vi "StepRealtime_IP6.vi"() -> ()   [LabVIEW 2011]
doc: "This VI was generated automatically using the FPGA Wizard. You can modify the VI normally."
uses:
  <vilib>/Platform/TimedLoop/XDataNode/timing_clust.ctl
  <vilib>/Platform/TimedLoop/XDataNode/nitl_modes.ctl
  <vilib>/Platform/TimedLoop/XDataNode/wakeup.ctl
  <vilib>/FPGAPlugInAG/sbRIO-9632/niLvFpga_Open_sbRIO-9632.vi
  <vilib>/rvi/interface/common/dynamic/niFpgaDynamicAddResources.vi
  <vilib>/FPGAPlugInAG/Dynamic/niLvFpga_Reset_Dynamic.vi
  <vilib>/FPGAPlugInAG/Dynamic/niLvFpga_Run_Dynamic.vi
  <vilib>/Utility/error.llb/Error Cluster From Error Code.vi
  <vilib>/rvi/errors/niLvFpgaAdjustHostInterfaceError.vi
  <vilib>/FPGAPlugInAG/Dynamic/niLvFpga_Close_Dynamic.vi
  <vilib>/rvi/interface/nirviOpenFPGA/nirviOpenFPGA.xnode
  FPGA Bitfiles/PPDControlLab3_FPGATarget_IP6.lvbitx
  <vilib>/rvi/interface/nirviMethod/nirviMethod.xnode
  <vilib>/Platform/TimedLoop/XDataNode/XDataNode.xnode
  <vilib>/rvi/interface/nirviReadWriteControl/nirviReadWriteControl.xnode
  <vilib>/rvi/interface/nirviCloseFPGA/nirviCloseFPGA.xnode
  SysIDRealtime.lvlib
  <vilib>/rvi/interface/Simulation/niFpgaSimulationCallBeginRW.vi
  <vilib>/Platform/TimedLoop/XDataNode/XDNodeRunTimeDep.lvlib
  NiFpgaLv.dll
panel:
  out "Ratio":fxp<+/-,32,7>
  in  "Gain":fxp<+/-,32,7>=0.006999999284744263
  in  "Radio Buttons":enum32{"Radio Selection 1", "Radio Selection 2"}(radio)
  in  "OK Button":bool
  out "Step Response":dynamicdata(graph)=[{"t0"=timestamp(0 s since 1904-01-01), "dt"=1.0, "Y"=array[2048 elements]}, {"t0"=timestamp(0 s since 1904-01-01), "dt"=1.0, "Y"=array[2048 elements]}, {"t0"=timestamp(0 s since 1904-01-01), "dt"=1.0, "Y"=array[2048 elements]}]
  in  "samples":i32=2048
  in  "Reference":i32=100000
  in  "Quad Reset":bool=TRUE
  in  "DGain":fxp<+/-,32,7>
  in  "PGain":fxp<+/-,32,7>
  out "Amp In":dbl[](graph)
  out "Amp Cpmmand":fxp<+/-,20,5>
  out "Iteration Duration":i64
  out "Position":i32[](graph)
  in  "Control Rate (ticks)":u32=10000
  in  "Period (us)":i64=1000
  out "Finished Late? [i-1]":bool
  out "quad saved (Port0/DIO0,Port0/DIO1)":cluster{"Position":i32, "Index Count":u16}
  out "quad pos (Port0/DIO0,Port0/DIO1)":i32
  out "Late? Latched":bool
  in  "Local Stop 0":bool
  in  "Start 0":bool
  in  "Loop Rate (Hz)":dbl=100000.0
  out "Calculated Rate (Hz)":dbl
  out "error out":errorcluster
  in  "Global Stop":bool
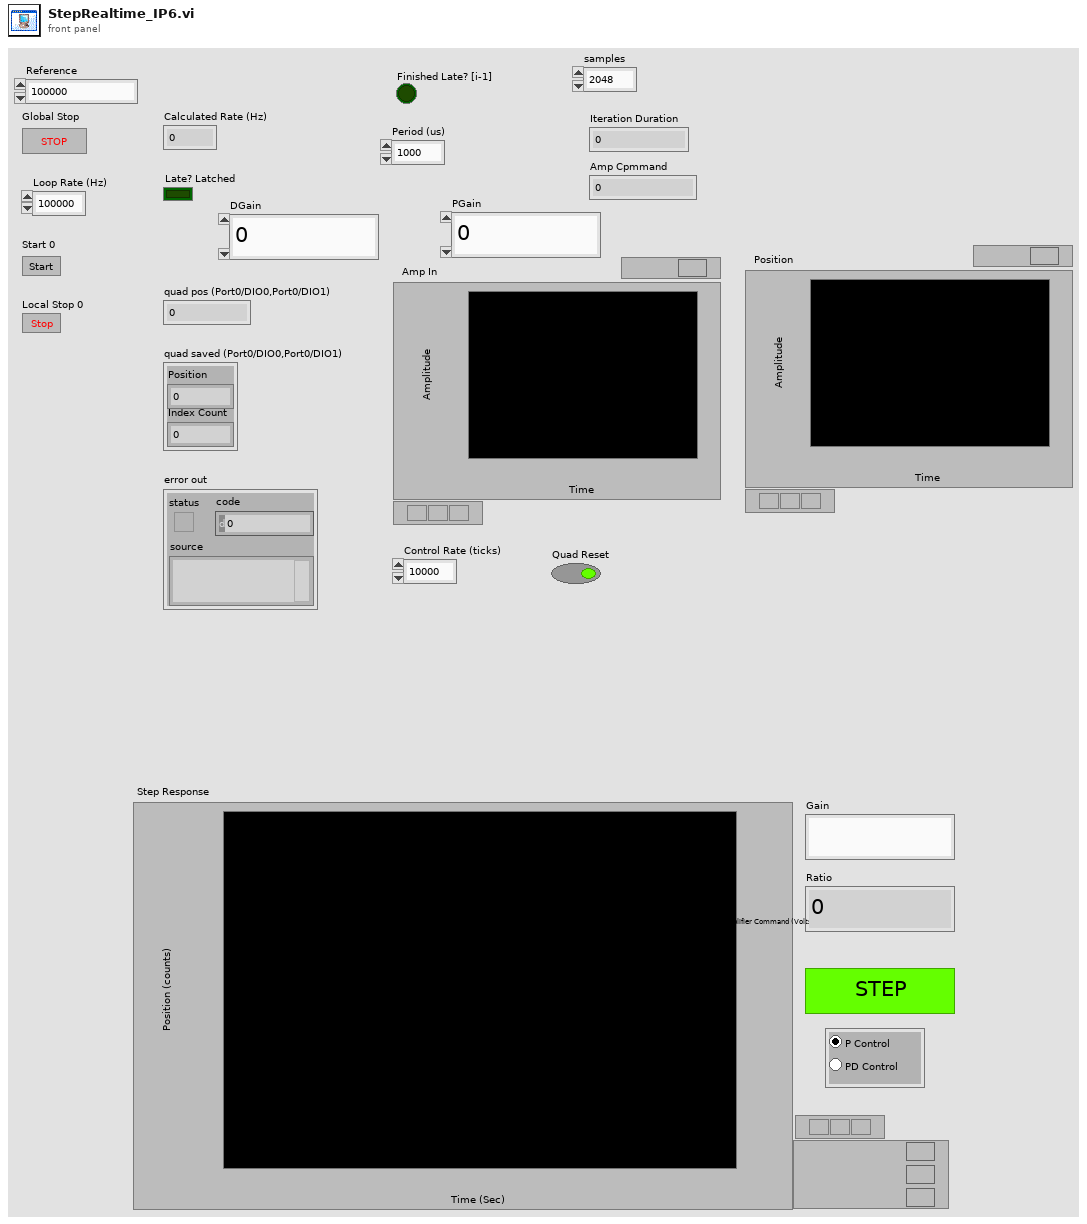
[diagram p1: front panel]
types:
  T1 = typedef "XDNodeRunTimeDep.lvlib/timing_clust.ctl" = cluster{"Expected End [f-1]":u64, "Actual End [f-1]":u64, "Finished Late? [f-1]":bool, "Expected End [i-1]":u64, "Actual End [i-1]":u64, "Finished Late? [i-1]":bool, "Expected Start [i]":u64, "Actual Start [i]":u64, "Expected Start [f]":u64, "Actual Start [f]":u64, "Source Name":string, "Structure Name":string, "Period":i64, "Deadline":i64, "Offset":i64, "Start":i64, "Priority":i32, "Timeout":i32, "Mode":T2, "Wakeup Reason":T3, "Error":errorcluster, "Source Type":string, "Secondary Source Type":string, "Global End Time":u64, "Global Start Time":u64, "Frame Duration":u64, "Iteration Duration":u64, "Assigned CPU":i32, "I/O Scan Engine Mode":u32}
  T2 = typedef "XDNodeRunTimeDep.lvlib/nitl_modes.ctl" = enum32{"No Change", "Process missed periods, maintain original phase", "Discard missed periods, maintain original phase", "Process missed periods, ignore original phase", "Discard missed periods, ignore original phase"}
  T3 = typedef "XDNodeRunTimeDep.lvlib/wakeup.ctl" = enum32{"Normal", "Aborted", "Asynchronous wakeup", "Timing source error", "Timed loop error", "Timeout"}
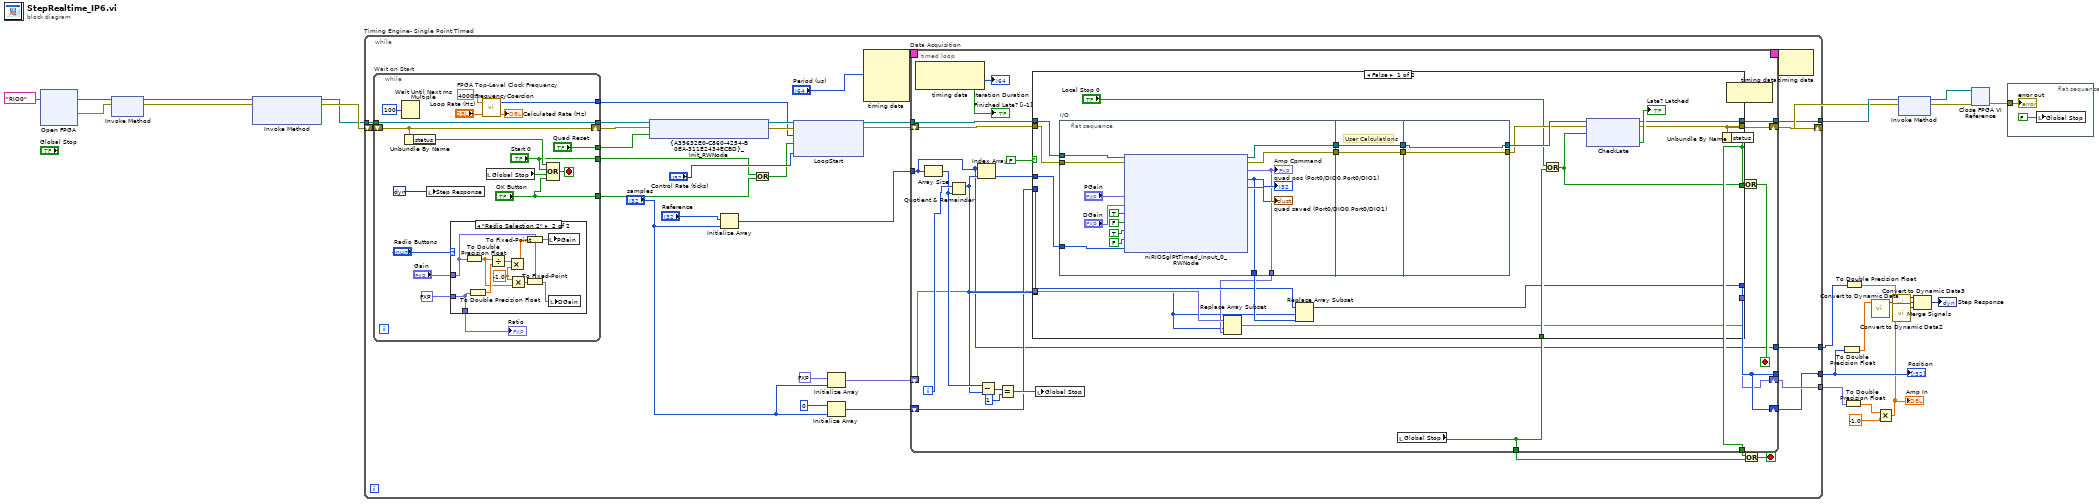
[diagram p0: block diagram]
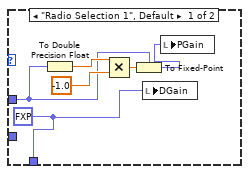
[diagram p3: hidden frame]
diagram:
  n1 = xnode ("Open FPGA")("resource name"=tag "RIO0") -> ("FPGA VI Reference Out"=w22:refnum<k20>, "error out"=w23:errorcluster)  [unwired: 1 in]
  n2 = xnode ("Invoke Method")("FPGA VI Reference In"=w22, "error in"=w23) -> ("FPGA VI Reference Out"=w5:refnum<k20>, "error out"=w4:errorcluster)
  n3 = xnode ("Invoke Method")("FPGA VI Reference In"=w5, "error in"=w4) -> ("FPGA VI Reference Out"=w10:refnum<k20>, "error out"=w24:errorcluster)  [unwired: 1 in]
  n4 = while "Timing Engine- Single Point Timed" {
    tunnel: w10 -> [w53]
    shift-right: [w52] -> w8
    shift-left: w24 -> [w56]
    tunnel: [w34] -> w16
    tunnel: [w35] -> w20
    tunnel: [w29] -> w14
    tunnel: [w25] -> w9
    stop <- w47 stop-if-true
    n5 = while "Wait on Start" {
      tunnel: w53 -> [w147]
      tunnel: [w147] -> w51
      tunnel: [w139] -> w44
      tunnel: ["Start 0"] -> w28
      shift-right: [w141] -> w50
      shift-left: w56 -> [w141]
      tunnel: ["Quad Reset"] -> w33
      tunnel: ["OK Button"] -> w27
      stop <- w148 stop-if-true
      w142 = 40000000.0  # FPGA Top-Level Clock Frequency
      n6 = Wait Until Next ms Multiple(millisecond multiple=u32 100) -> ()  [unwired: 1 out]
      n7 = Unbundle By Name(w141) -> ("status"=w140:bool)
      n8 = local write "Step Response"(dynamicdata [] ("Step Response")) -> ()
      n9 = case shown="\"Radio Selection 2\"" "Radio Buttons" {
        tunnel: "Gain" -> [w150 w156]
        tunnel: fxp<+/-,32,7> 40.0 ("Ratio") -> [_ w161]
        tunnel: [w154 w161] -> w132
        frame "Radio Selection 1", Default {
          w154 = fxp<+/-,32,7> 0.0 ("DGain")
          n10 = To Double Precision Float(number=w150) -> (double precision float=w153:dbl)
          n11 = Multiply(x=w153, y=-1.0) -> (x*y=w151:dbl)
          n12 = To Fixed-Point(fixed-point type=w150, number=w151) -> (fixed-point=w149:fxp<+/-,32,7>)
          n13 = local write "DGain"(w154) -> ()
          n14 = local write "PGain"(w149) -> ()
        }
        frame "Radio Selection 2" {
          w159 = -1.0 ("y")
          n15 = To Double Precision Float(number=w156) -> (double precision float=w158:dbl)
          n16 = To Double Precision Float(number=w161) -> (double precision float=w164:dbl)
          n17 = Divide(x=w158, y=w164) -> (x/y=w163:dbl)
          n18 = Multiply(x=w163, y=w159) -> (x*y=w160:dbl)
          n19 = Multiply(x=w159, y=w158) -> (x*y=w157:dbl)
          n20 = To Fixed-Point(fixed-point type=w156, number=w160) -> (fixed-point=w162:fxp<+/-,32,7>)
          n21 = To Fixed-Point(fixed-point type=w156, number=w157) -> (fixed-point=w155:fxp<+/-,32,7>)
          n22 = local write "PGain"(w162) -> ()
          n23 = local write "DGain"(w155) -> ()
        }
      }
      "Ratio" <- w132
      n24 = call "FrequencyCoercion.vi"("Loop Rate (Hz)"="Loop Rate (Hz)", "FPGA Top-Level Clock Frequency"=w142) -> ("Actual Rate (Hz)"=→"Calculated Rate (Hz)":dbl, "FPGA Ticks"=w139:u32)  [unwired: 2 in]
      n25 = local read "Global Stop"() -> (w145:bool)
      n26 = Compound Arithmetic op=OR(w140, "Start 0", w145, "OK Button") -> (w148:bool)
    }
    n27 = xnode ("{A39632E0-C860-4254-B0EA-311E2434ECBD}_Init_RWNode")("FPGA VI Reference In"=w51, "error in"=w50, "quad reset (Port0/DIO0,Port0/DIO1)"=w33) -> ("FPGA VI Reference Out"=w45:refnum<k20>, "error out"=w49:errorcluster)
    n28 = Initialize Array("Reference", "samples") -> (w30:i32[])
    n29 = Or(x=w28, y=w27) -> (x .or. y?=w26:bool)
    n30 = xnode ("LoopStart")("FPGA VI Reference In"=w45, "error in"=w49, "Loop Rate (Ticks)"=w44, "Start 0"=w26, "Control Rate (ticks)"="Control Rate (ticks)") -> ("FPGA VI Reference Out"=w55:refnum<k20>, "error out"=w54:errorcluster)
    n31 = Initialize Array(0 ("quad pos (Port0/DIO0,Port0/DIO1)"), "samples") -> (w38:i32[])
    n32 = Initialize Array(fxp<+/-,20,5> 0.0 ("Amp Cpmmand"), "samples") -> (w36:fxp<+/-,20,5>[])
    n33 = node-c288("Period (us)") -> (w43:T1)  [unwired: 3 in]
    n34 = timed-loop "Data Acquisition" {
      tunnel: w55 -> [w74]
      tunnel: [w76] -> w48
      tunnel: [w75] -> w46
      shift-right: [w79] -> w52
      shift-left: w54 -> [w73]
      timing: w43 -> [_]
      timing-out: [_] -> w42
      tunnel: w30 -> [w58]
      tunnel: [w60] -> _
      shift-right: [w59] -> w35
      shift-left: w36 -> [w61]
      shift-right: [w60] -> w34
      shift-left: w38 -> [w63]
      tunnel: [w58] -> w29
      tunnel: [w57] -> w25
      i -> [w70]
      stop <- w77 stop-if-true
      n35 = node-c288() -> (→"Finished Late? [i-1]":bool, →"Iteration Duration":i64)  [unwired: 1 in]
      n36 = Array Size(array=w58) -> (size(s)=w68:i32)
      n37 = Quotient & Remainder(x=w70, y=w68) -> (x-y*floor(x/y)=w64:i32)  [unwired: 1 out]
      n38 = Index Array(array=w58, index=w64) -> (element=w69:i32)
      n39 = Subtract(x=w68, y=w64) -> (x-y=w67:i32)
      n40 = Equal?(x=w67, y=1) -> (x = y?=w65:bool)
      n41 = local write "Global Stop"(w65) -> ()
      n42 = local read "Global Stop"() -> (w76:bool)
      n43 = case "Timeout" shown="False" FALSE {
        tunnel: w74 -> [w100 w124]
        tunnel: w73 -> [w99 w126]
        tunnel: [w93 w126] -> w79
        tunnel: [w95 w125] -> w78
        tunnel: w76 -> [w96 w125]
        tunnel: w69 -> [w85 _]
        tunnel: w64 -> [w87 _]
        tunnel: w63 -> [w91 _]
        tunnel: [w90 _] -> w60
        tunnel: w61 -> [w89 _]
        tunnel: [w86 _] -> w59
        tunnel: [w84 w124] -> w57
        frame False {
          n44 = flat-sequence "I/O" {
            tunnel: w100 -> [w117]
            tunnel: w99 -> [w119]
            tunnel: [w118] -> w105
            tunnel: [w116] -> w102
            tunnel: [w114] -> w92
            tunnel: [w113] -> w88
            tunnel: w85 -> [w106]
            tunnel: [w121] -> w104
            tunnel: w105 -> [w120]
            tunnel: w102 -> [w121]
            tunnel: [w120] -> w103
            tunnel: [w122] -> w98
            tunnel: [w123] -> w101
            tunnel: w104 -> [w123]
            tunnel: w103 -> [w122]
            frame #0 {
              n45 = xnode ("niRIOSglPtTimed_Input_0_RWNode")("FPGA VI Reference In"=w117, "error in"=w119, "PGain"="PGain", "DGain"="DGain", "Amp Enable"=TRUE, "Amp Reset"=FALSE, "Brake"=TRUE, "quad reset (Port0/DIO0,Port0/DIO1)"=FALSE, "Reference"=w106) -> ("FPGA VI Reference Out"=w116:refnum<k20>, "error out"=w118:errorcluster, "Amp Cpmmand"=w113:fxp<+/-,20,5>, "quad pos (Port0/DIO0,Port0/DIO1)"=w114:i32, "quad saved (Port0/DIO0,Port0/DIO1)"=→"quad saved (Port0/DIO0,Port0/DIO1)":cluster{"Position":i32, "Index Count":u16})
              "quad pos (Port0/DIO0,Port0/DIO1)" <- w114
              "Amp Cpmmand" <- w113
            }
            frame #1 {
              # "User Calculations"
            }
            frame #2 {
            }
          }
          n46 = Replace Array Subset(array=w89, new element=w88, index=w87) -> (w86:fxp<+/-,20,5>[])
          n47 = Replace Array Subset(array=w91, new element=w92, index=w87) -> (w90:i32[])
          n48 = Or(x="Local Stop 0", y=w96) -> (x .or. y?=w95:bool)
          n49 = xnode ("CheckLate")("FPGA VI Reference In"=w101, "error in"=w98, "Local Stop 0"=w95) -> ("FPGA VI Reference Out"=w84:refnum<k20>, "error out"=w93:errorcluster, "Late? Latched"=→"Late? Latched":bool)
        }
        frame True {
          # "Timeout waiting for an interrupt. This case checks the state of the global stop.\nIf global stop is not set, then loop around to wait for an interrupt again."
        }
      }
      n50 = Unbundle By Name(w79) -> ("status"=w75:bool)
      n51 = node-c288() -> ()  [unwired: 1 in, 1 out]
      n52 = Or(x=w75, y=w78) -> (x .or. y?=w77:bool)
    }
    n53 = Or(x=w46, y=w48) -> (x .or. y?=w47:bool)
    n54 = node-c288(w42) -> ()  [unwired: 1 out]
  }
  "Position" <- w16
  n55 = To Double Precision Float(number=w16) -> (double precision float=w15:dbl[])
  n56 = To Double Precision Float(number=w20) -> (double precision float=w2:dbl[])
  n57 = To Double Precision Float(number=w14) -> (double precision float=w13:dbl[])
  n58 = call "Convert to Dynamic Data"("Array"=w15) -> ("Dynamic Data Type"=w18:dynamicdata)  [unwired: 3 in]
  n59 = Multiply(x=w2, y=-1.0) -> (x*y=w1:dbl[])
  "Amp In" <- w1
  n60 = call "Convert to Dynamic Data3"("Array"=w13) -> ("Dynamic Data Type"=w12:dynamicdata)  [unwired: 3 in]
  n61 = call "Convert to Dynamic Data2"("Array"=w1) -> ("Dynamic Data Type"=w17:dynamicdata)  [unwired: 3 in]
  n62 = xnode "Invoke Method"("FPGA VI Reference In"=w9, "error in"=w8) -> ("FPGA VI Reference Out"=w7:refnum<k20>, "error out"=w6:errorcluster)
  n63 = Merge Signals(w12, w18, w17) -> (→"Step Response":dynamicdata)
  n64 = xnode ("Close FPGA VI Reference")("FPGA VI Reference In"=w7, "error in"=w6) -> ("error out"=w21:errorcluster)
  n65 = flat-sequence {
    tunnel: w21 -> [w166]
    frame #0 {
      n66 = local write "Global Stop"(FALSE ("Global Stop")) -> ()
      "error out" <- w166
    }
  }
